vi "Stop SSH Client.vi"(11 "Module Data":T1) -> (0 "error out":errorcluster)   [LabVIEW 2017, in "SSH.lvlib"]
uses:
  SSH.lvlib
  Module Data--cluster.ctl
  C:/Users/phorn/Documents/LV_SSH/Renci.SshNet.dll
  Renci.SshNet.dll
  Response Configuration.ctl
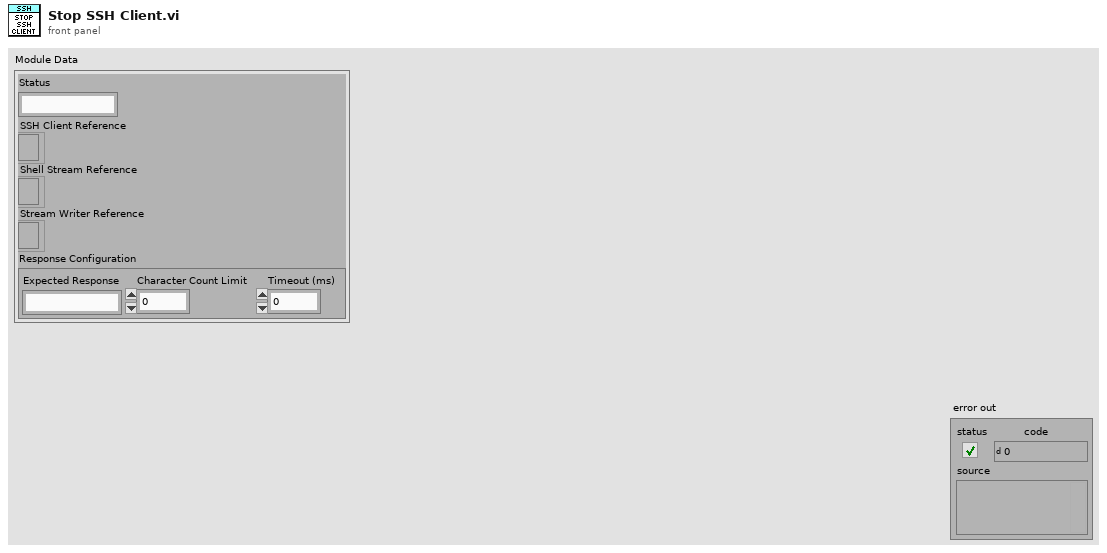
[diagram p1: front panel]
types:
  T1 = typedef "SSH.lvlib/Module Data--cluster.ctl" = cluster{"Status":string, "SSH Client Reference":refnum<k24>, "Shell Stream Reference":refnum<k24>, "Stream Writer Reference":refnum<k24>, "Response Configuration":T2}
  T2 = typedef "Response Configuration.ctl" = cluster{"Expected Response":string, "Character Count Limit":dbl, "Timeout (ms)":dbl}
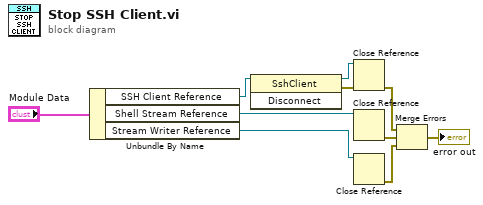
[diagram p0: block diagram]
diagram:
  n1 = Unbundle By Name("Module Data") -> ("SSH Client Reference"=w9:refnum<k24>, "Shell Stream Reference"=w8:refnum<k24>, "Stream Writer Reference"=w7:refnum<k24>)
  n2 = invoke class="SshClient" method="Disconnect"(reference=w9) -> (reference out=w6:refnum<k24>, error out=w5:errorcluster)  [unwired: 2 in, 1 out]
  n3 = Close Reference(reference=w6, error in (no error)=w5) -> (error out=w4:errorcluster)
  n4 = Close Reference(reference=w8) -> (error out=w3:errorcluster)  [unwired: 1 in]
  n5 = Close Reference(reference=w7) -> (error out=w2:errorcluster)  [unwired: 1 in]
  n6 = Merge Errors(w4, w3, w2) -> (→"error out":errorcluster)
